vi "Get Wavelength.vi"(8 "error in (no error)":errorcluster, 11 "Topas in":refnum<class "Topas3.lvclass">) -> (0 "error out":errorcluster, 2 "Wavelength":dbl, 3 "Topas out":refnum<class "Topas3.lvclass">)   [LabVIEW 2020, in "Topas3.lvclass"]
uses:
  Topas3.lvclass
  Topas3.lvclass/Topas3.ctl
  Topas-LabVIEW-Driver/TopasDriver.lvlib
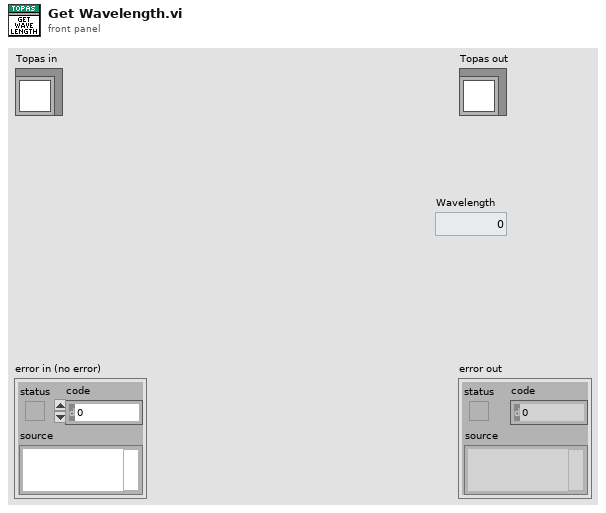
[diagram p1: front panel]
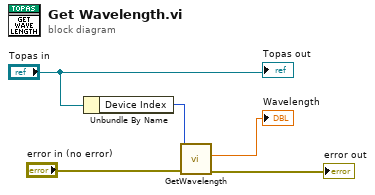
[diagram p0: block diagram]
diagram:
  n1 = Unbundle By Name("Topas in") -> ("Device Index"=w1:u8)
  n2 = call "GetWavelength.vi"("error in (no error)"="error in (no error)", "Device Index"=w1) -> ("error out"=→"error out":errorcluster, "Wavelength"=→"Wavelength":dbl)  [unwired: 6 in, 2 out]
  "Topas out" <- "Topas in"
